vi "Agilent VNA Format String with Channel and Trace.vi"(4 "Trace":i8=1 min=1 max=99 step=1, 5 "Channel":i8=1 min=1 max=99 step=1, 8 "String":string) -> (2 "String Out":string)   [LabVIEW 2011]
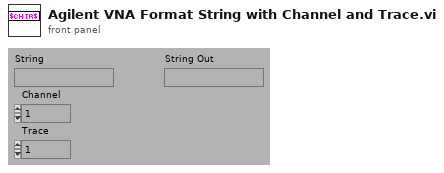
[diagram p1: front panel]
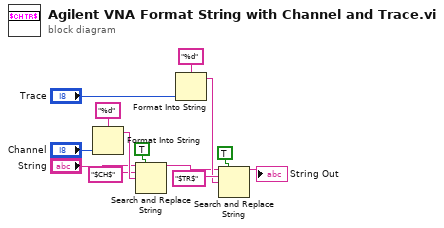
[diagram p0: block diagram]
diagram:
  n1 = Format Into String(format string="%d", "Channel") -> (resulting string=w13:string)  [unwired: 2 in, 1 out]
  n2 = Search and Replace String(replace all?=TRUE ("replace all? (F)"), input string="String", search string="$CH$", replace string=w13) -> (result string=w2:string)  [unwired: 1 in, 6 out]
  n3 = Format Into String(format string="%d", "Trace") -> (resulting string=w4:string)  [unwired: 2 in, 1 out]
  n4 = Search and Replace String(replace all?=TRUE ("replace all? (F)"), input string=w2, search string="$TR$", replace string=w4) -> (result string=→"String Out":string)  [unwired: 1 in, 6 out]
